vi "Complex to DB.vi"(8 "error in (no error)":errorcluster, 11 "Complex Data In":refnum<class "2D Array c32.lvclass">) -> (0 "error out":errorcluster, 3 "Amplitude dB Out":refnum<class "2D Array f32.lvclass">)   [LabVIEW 2020, in "GPU FFT Calculator.lvlib" / "GPU FFT Calculator.lvclass"]
uses:
  GPU FFT Calculator.lvclass
  <vilib>/Natan Biesmans/G2CPU GPU and CPU HPC Toolkit/G2CPU Libraries/Arrays/2DArray/f32/2D Array f32.lvclass
  C:/Program Files/National Instruments/LabVIEW 2026/vi.lib/Natan Biesmans/G2CPU GPU and CPU HPC Toolkit/G2CPU Libraries/Arrays/Array/Array Prototype.lvclass
  <vilib>/Natan Biesmans/G2CPU GPU and CPU HPC Toolkit/G2CPU Libraries/Arrays/2DArray/c32/2D Array c32.lvclass
  <vilib>/Natan Biesmans/G2CPU GPU and CPU HPC Toolkit/G2CPU Libraries/Arrays/Array/Array Prototype.lvclass/Array Prototype.ctl
  4621f685-081b-4daf-8f60-e6de4fc88aa0.vi
  9a73ff79-72b4-4811-bfe7-b1b640eba118.vi
  e5b434b2-97c5-432c-b0c5-545dc51e6fe8.vi
  1348d077-7cad-4560-bf5b-1b7c29b7c389.vi
  <vilib>/Natan Biesmans/G2CPU GPU and CPU HPC Toolkit/G2CPU Libraries/Arrays/Array/G2CPU Get Array Pointer.vi
  4621f685-081b-4daf-8f60-e6de4fc88aa0.vi/b6535cc3-4f5d-45ad-9052-c08cd62b0315.vi
  <vilib>/Natan Biesmans/G2CPU GPU and CPU HPC Toolkit/ArrayFire Driver/VIs/release array.vi
  4621f685-081b-4daf-8f60-e6de4fc88aa0.vi/c9d07b13-7729-4cda-a81e-7ca6043257da.vi
  4621f685-081b-4daf-8f60-e6de4fc88aa0.vi/4470c8c9-d353-49e9-bc1e-f4fe0b2204ee.vi
  4621f685-081b-4daf-8f60-e6de4fc88aa0.vi/b48f0110-6046-499d-b6aa-1db73cdea65c.vi
  9a73ff79-72b4-4811-bfe7-b1b640eba118.vi/def40612-844c-421c-bb75-87c330777b0b.vi
  e5b434b2-97c5-432c-b0c5-545dc51e6fe8.vi/31b317ac-79b4-42cb-9c55-b9b94a2bc574.vi
  1348d077-7cad-4560-bf5b-1b7c29b7c389.vi/6197f869-f6d4-49b3-9b2c-cc979b422c2e.vi
  1348d077-7cad-4560-bf5b-1b7c29b7c389.vi/a7e86dbb-b4c0-485c-89c5-522e60ee265c.vi
  <vilib>/Natan Biesmans/G2CPU GPU and CPU HPC Toolkit/ArrayFire Driver/VIs/Run as Multi Device.vi
  <vilib>/Natan Biesmans/G2CPU GPU and CPU HPC Toolkit/G2CPU Libraries/Runtime Licensing/G2CPU License Check.vi
  1348d077-7cad-4560-bf5b-1b7c29b7c389.vi/6197f869-f6d4-49b3-9b2c-cc979b422c2e.vi/3e802c67-fb96-46a3-ae13-4994a8508b4f.vi
  1348d077-7cad-4560-bf5b-1b7c29b7c389.vi/6197f869-f6d4-49b3-9b2c-cc979b422c2e.vi/5a50fc67-79e7-4972-80c2-92243cd53dd4.vi
  1348d077-7cad-4560-bf5b-1b7c29b7c389.vi/6197f869-f6d4-49b3-9b2c-cc979b422c2e.vi/4b7910ad-0c4a-46e4-b1b3-c9721aeaa91e.vi
  1348d077-7cad-4560-bf5b-1b7c29b7c389.vi/a7e86dbb-b4c0-485c-89c5-522e60ee265c.vi/730f6c57-5c0b-4ee9-b61e-75067b25222b.vi
  1348d077-7cad-4560-bf5b-1b7c29b7c389.vi/a7e86dbb-b4c0-485c-89c5-522e60ee265c.vi/096b8799-7810-404e-baca-ba9279cec4bd.vi
  1348d077-7cad-4560-bf5b-1b7c29b7c389.vi/a7e86dbb-b4c0-485c-89c5-522e60ee265c.vi/0f1a5a47-bcc5-4796-ac31-8dfcfbc0d7d1.vi
  1348d077-7cad-4560-bf5b-1b7c29b7c389.vi/a7e86dbb-b4c0-485c-89c5-522e60ee265c.vi/89f12e17-3330-4b72-ad8f-8dd636660732.vi
  1348d077-7cad-4560-bf5b-1b7c29b7c389.vi/6197f869-f6d4-49b3-9b2c-cc979b422c2e.vi/5a50fc67-79e7-4972-80c2-92243cd53dd4.vi/1b7cf390-2ae0-48f3-9bce-03c57eed6ee8.vi
  1348d077-7cad-4560-bf5b-1b7c29b7c389.vi/a7e86dbb-b4c0-485c-89c5-522e60ee265c.vi/730f6c57-5c0b-4ee9-b61e-75067b25222b.vi/0070e0fe-4ad7-4a3e-8965-d64becb7e5f0.vi
  <vilib>/Natan Biesmans/G2CPU GPU and CPU HPC Toolkit/G2CPU Libraries/Arrays/1DArray/f32/1D Array f32.lvclass
  <vilib>/Natan Biesmans/G2CPU GPU and CPU HPC Toolkit/ArrayFire Driver/VIs/real.vi
  <vilib>/Natan Biesmans/G2CPU GPU and CPU HPC Toolkit/ArrayFire Driver/VIs/imag.vi
  <vilib>/Natan Biesmans/G2CPU GPU and CPU HPC Toolkit/ArrayFire Driver/VIs/hypot.vi
  <vilib>/Natan Biesmans/G2CPU GPU and CPU HPC Toolkit/G2CPU Libraries/Arrays/SubVI/G2CPU State.vi
  <vilib>/NI License Manager/Open Session.vi
  <vilib>/NI License Manager/Check License Status.vi
  <vilib>/NI License Manager/Check License Status (Single).vi
  <vilib>/NI License Manager/Activate License.vi
  <vilib>/NI License Manager/Activate License (Single).vi
  <vilib>/NI License Manager/Close Session.vi
  <vilib>/Natan Biesmans/G2CPU GPU and CPU HPC Toolkit/ArrayFire Driver/subvi/Error Converter (ErrCode or Status).vi
  <vilib>/Natan Biesmans/G2CPU GPU and CPU HPC Toolkit/ArrayFire Driver/VIs/arg.vi
  <vilib>/Natan Biesmans/G2CPU GPU and CPU HPC Toolkit/G2CPU Libraries/Arrays/Array/G2CPU Set Array Pointer.vi
  <vilib>/Natan Biesmans/G2CPU GPU and CPU HPC Toolkit/ArrayFire Driver/VIs/abs.vi
  <vilib>/Natan Biesmans/G2CPU GPU and CPU HPC Toolkit/ArrayFire Driver/VIs/log10.vi
  <vilib>/Natan Biesmans/G2CPU GPU and CPU HPC Toolkit/G2CPU Libraries/Arrays/SubVI/is 2D.vi
  <vilib>/Natan Biesmans/G2CPU GPU and CPU HPC Toolkit/ArrayFire Driver/VIs/mul.vi
  <vilib>/Natan Biesmans/G2CPU GPU and CPU HPC Toolkit/G2CPU Libraries/Arrays/Array/Array Prototype.lvclass
  <vilib>/Natan Biesmans/G2CPU GPU and CPU HPC Toolkit/G2CPU Libraries/Arrays/DataTypes/c32/c32.lvclass
  <vilib>/Natan Biesmans/G2CPU GPU and CPU HPC Toolkit/G2CPU Libraries/Arrays/2DArray/2D Array Prototype.lvclass
  <vilib>/Natan Biesmans/G2CPU GPU and CPU HPC Toolkit/G2CPU Libraries/Arrays/DataTypes/f32/f32.lvclass
  <vilib>/Natan Biesmans/G2CPU GPU and CPU HPC Toolkit/G2CPU Libraries/Arrays/1DArray/1D Array Prototype.lvclass
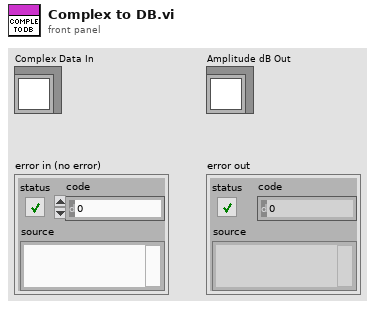
[diagram p1: front panel]
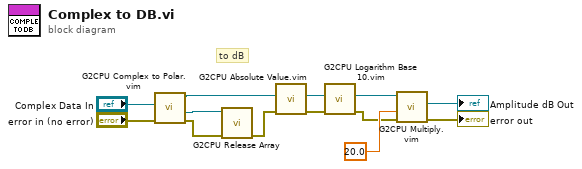
[diagram p0: block diagram]
diagram:
  # "to dB"
  n1 = call "G2CPU Complex to Polar.vim"("error in (no error)"="error in (no error)", "Array Real"="Complex Data In") -> ("error out"=w11:errorcluster, "Array Theta"=w10:refnum<class "2D Array f32.lvclass">, "Array r"=w9:refnum<class "2D Array f32.lvclass">)  [unwired: 7 in]
  n2 = call-dynamic "G2CPU Release Array.vi"("error in (no error)"=w11, "Array in"=w10) -> ("error out"=w1:errorcluster)  [unwired: 9 in]
  n3 = call "G2CPU Absolute Value.vim"("error in (no error)"=w1, "Array in"=w9) -> ("error out"=w3:errorcluster, "Array Result"=w2:refnum<class "2D Array f32.lvclass">)  [unwired: 8 in]
  n4 = call "G2CPU Logarithm Base 10.vim"("error in (no error)"=w3, "Array in"=w2) -> ("error out"=w5:errorcluster, "Array Result"=w4:refnum<class "2D Array f32.lvclass">)  [unwired: 8 in]
  n5 = call "G2CPU Multiply.vim"("error in (no error)"=w5, "Array rhs"=sgl 20.0, "Array lhs"=w4) -> ("error out"=→"error out":errorcluster, "Array Result"=→"Amplitude dB Out":refnum<class "2D Array f32.lvclass">)  [unwired: 7 in]
